vi "题目五.vi"() -> ()   [LabVIEW 2017]
panel:
  out "显示面板":T1 {"油量" scale=0.0..200.0; "转速（r/s）" scale=0.0..8000.0; "速度（Km/h）" scale=0.0..300.0}
  in  "停止":bool
  out "油量报警":bool
  in  "控制面板":T2 {"档位" scale=0.0..10.0; "油门" scale=0.0..10.0}
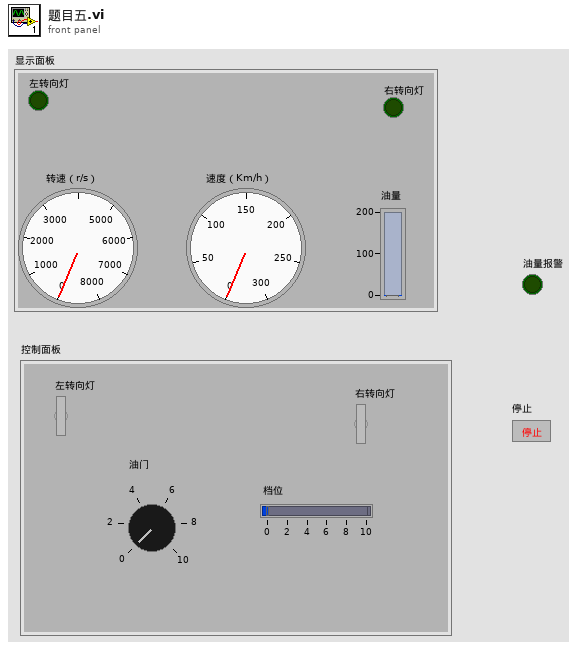
[diagram p1: front panel]
types:
  T1 = cluster{"左转向灯":bool, "右转向灯":bool, "转速（r/s）":dbl, "速度（Km/h）":dbl, "油量":dbl}
  T2 = cluster{"左转向灯":bool, "右转向灯":bool, "油门":dbl, "档位":dbl}
  T3 = cluster{"左转向灯":bool, "右转向灯":bool, dbl, dbl, "b":dbl}
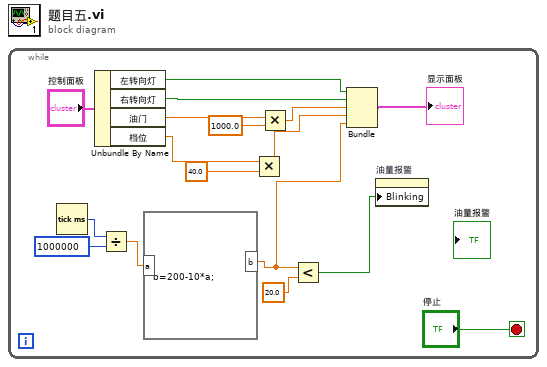
[diagram p0: block diagram]
diagram:
  n1 = while {
    stop <- "停止" stop-if-true
    n2 = Tick Count (ms)() -> (millisecond timer value=w2:u32)
    n3 = Unbundle By Name("控制面板") -> ("左转向灯"=w16:bool, "右转向灯"=w5:bool, "油门"=w15:dbl, "档位"=w12:dbl)
    n4 = Divide(x=w2, y=u32 1000000) -> (x/y=w3:dbl)
    n5 = formula code="b=200-10*a;"("a"=w3) -> ("b"=w7:dbl)
    n6 = Multiply(x=w12, y=40.0) -> (x*y=w10:dbl)
    n7 = Multiply(x=w15, y=1000.0) -> (x*y=w13:dbl)
    n8 = Less?(x=w7, y=20.0) -> (x < y?=w6:bool)
    n9 = Bundle("左转向灯"=w16, "右转向灯"=w5, w13, w10, "b"=w7) -> (→"显示面板":T3)  [unwired: 1 in]
    n10 = property on="油量报警" class="Bool (严格)"("Blinking"=w6) -> ()  [unwired: 2 in, 2 out]
  }
